vi "createChildEvents.vi"(8 "error in (no error)":errorcluster, 11 "CommandEvents in":refnum<class "CommandEvents.lvclass">) -> (0 "error out":errorcluster, 3 "CommandEvents out":refnum<class "CommandEvents.lvclass">)   [LabVIEW 2011, in "Tools.lvlib" / "Interpreters.lvlib" / "CommandEvents.lvclass"]
uses:
  CommandEvents.lvclass
  CommandEvents.lvclass/CommandEvents.ctl
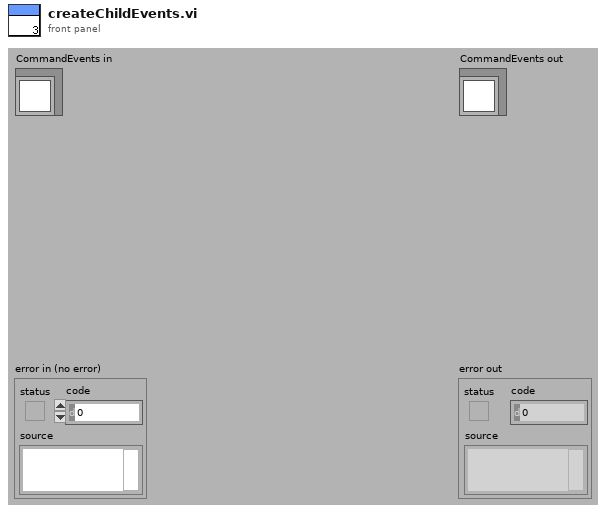
[diagram p1: front panel]
types:
  T1 = cluster{"newCommand":refnum<user-event>, "textUpdate":refnum<user-event>}
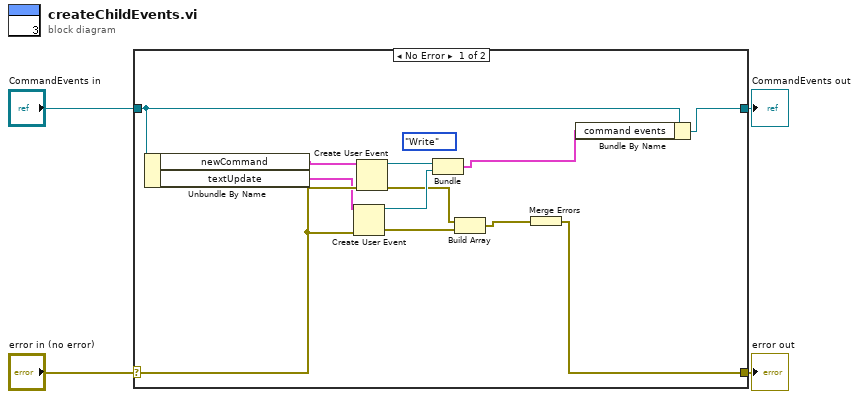
[diagram p0: block diagram]
diagram:
  n1 = case shown="No Error" "error in (no error)" {
    selector: "error in (no error)" -> [w14 w18]
    tunnel: [w8 w18] -> w3
    tunnel: [w6 w17] -> w1
    tunnel: "CommandEvents in" -> [w7 w17]
    frame No Error {
      (unwired) enum16{"Write", "Read"}."Write" ("Action")
      n2 = Unbundle By Name(w7) -> ("newCommand"=w16:cluster{"command":string}, "textUpdate"=w13:cluster{"updateText":string})
      n3 = Create User Event(user event datatype=w13, error in=w14) -> (user event=w12:refnum<user-event>, error out=w10:errorcluster)
      n4 = Create User Event(user event datatype=w16, error in=w14) -> (user event=w15:refnum<user-event>, error out=w11:errorcluster)
      n5 = Bundle("newCommand"=w15, "textUpdate"=w12) -> (w5:T1)  [unwired: 1 in]
      n6 = Build Array(w11, w10) -> (w9:errorcluster[])
      n7 = Merge Errors(w9) -> (w8:errorcluster)
      n8 = Bundle By Name(cluster=w7, "command events"=w5) -> (w6:refnum<class "CommandEvents.lvclass">)
    }
    frame Error {
    }
  }
  "error out" <- w3
  "CommandEvents out" <- w1
